vi "GIP CAN Main.vi"(8 "error in":errorcluster, 10 "Interface":refnum<k21>="CAN1") -> (0 "error out":errorcluster={"status"=TRUE, "code"=-1074384711, "source"="XNET Create Session (Signal Input Single-point).vi:6590002<APPEND>\n\n<b>Complete call chain:</b>\r\n     XNET Create Session (Signal Input Single-point).vi:6590002\r\n     CAN GIP.lvlib:GIP CAN Wrapper.vi:2150001\r\n     CAN GIP.lvlib:CAN GIP Test.vi"}, 3 "output":dbl[](array[numeric]))   [LabVIEW 2021, in "CAN GIP.lvlib"]
uses:
  CAN GIP.lvlib
  Private Controls/CAN States.ctl
  Private Controls/Setting.ctl
panel:
  in  "Tx Signal In":string
  in  "Signal Write":dbl
  in  "Tx":bool
  in  "stop":bool
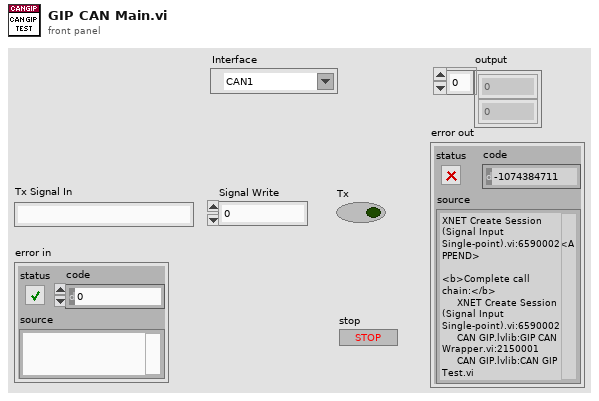
[diagram p1: front panel]
types:
  T1 = typedef "CAN GIP.lvlib/Setting.ctl" = cluster{"Termination":u32, "Baud Rate":u64, "Interface":refnum<k21>, "XNET Database":refnum<k21>, "ECU":refnum<k21>}
  T2 = typedef "CAN GIP.lvlib/CAN States.ctl" = enum16{"Init", "Config", "Read Signals", "Write Signals", "Close"}
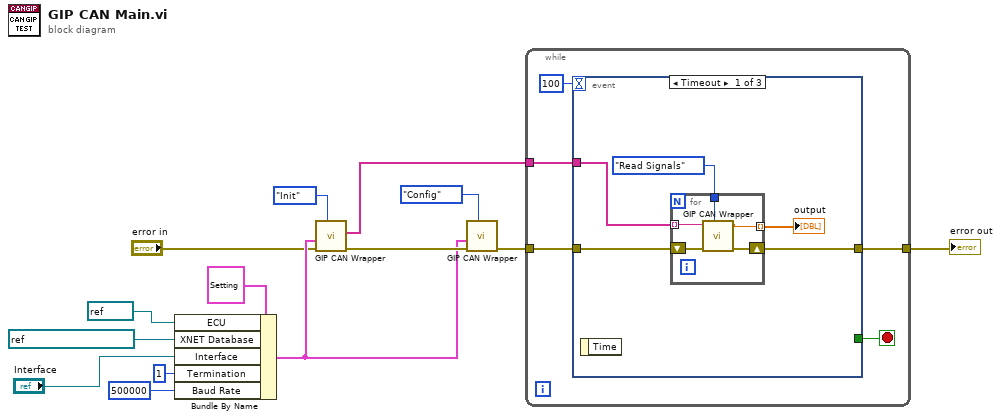
[diagram p0: block diagram]
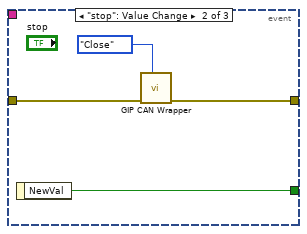
[diagram p2: hidden frame]
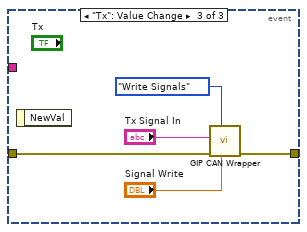
[diagram p3: hidden frame]
diagram:
  n1 = Bundle By Name(cluster=T1 {"Termination"=1, "Baud Rate"=125000, "Interface"="CAN1", "XNET Database"="GIP_CAN_Database", "ECU"="GIP\nGIP_CAN_Database"} ("Setting"), "ECU"=refnum<k21> "GIP\ncan_messages_818", "XNET Database"=refnum<k21> "can_messages_818", "Interface"="Interface", "Termination"=u32 1, "Baud Rate"=u64 500000) -> (w10:T1)
  n2 = call "GIP CAN Wrapper.vi"("States"=CAN_States."Init" ("CAN States"), "error in"="error in", "Setting"=w10) -> ("error out"=w13:errorcluster, "Rx SigNames"=w2:string[])  [unwired: 6 in, 1 out]
  n3 = call "GIP CAN Wrapper.vi"("States"=CAN_States."Config" ("CAN States"), "error in"=w13, "Setting"=w10) -> ("error out"=w9:errorcluster)  [unwired: 6 in, 2 out]
  n4 = while {
    tunnel: [w15] -> w1
    tunnel: w9 -> [w17]
    tunnel: w2 -> [w16]
    stop <- w18 stop-if-true
    n5 = event shown="[0] Timeout" {
      selector: _ -> [_ _ _]
      dyn-events: _ -> [_ _ _]
      timeout: 100 -> [_ _ _]
      tunnel: [_ w33 _] -> w18
      tunnel: w17 -> [w22 w31 w37]
      tunnel: w16 -> [w20 _ _]
      tunnel: [w21 w30 w36] -> w15
      event Timeout {
        n6 = event-data() -> ()  [unwired: 1 in, 1 out]
        n7 = for {
          tunnel: CAN_States."Read Signals" ("CAN States") -> [w29]
          tunnel: w20 -> [w27] mode=indexing
          shift-right: [w26] -> w21
          shift-left: w22 -> [w28]
          tunnel: [w25] -> w24 mode=indexing
          n8 = call "GIP CAN Wrapper.vi"("States"=w29, "error in"=w28, "Rx Signal In"=w27) -> ("error out"=w26:errorcluster, "Signal out"=w25:dbl)  [unwired: 6 in, 1 out]
        }
        "output" <- w24
      }
      event "stop": Value Change {
        n9 = event-data() -> ("NewVal"=w33:bool)  [unwired: 1 in]
        n10 = call "GIP CAN Wrapper.vi"("States"=CAN_States."Close" ("CAN States"), "error in"=w31) -> ("error out"=w30:errorcluster)  [unwired: 7 in, 2 out]
      }
      event "Tx": Value Change {
        n11 = event-data() -> ()  [unwired: 1 in, 1 out]
        n12 = call "GIP CAN Wrapper.vi"("Signal Write"="Signal Write", "States"=CAN_States."Write Signals" ("CAN States"), "error in"=w37, "Tx Signal In"="Tx Signal In") -> ("error out"=w36:errorcluster)  [unwired: 5 in, 2 out]
      }
    }
  }
  "error out" <- w1
